vi "Case Structure Tunnels.vi"   [LabVIEW 2015]
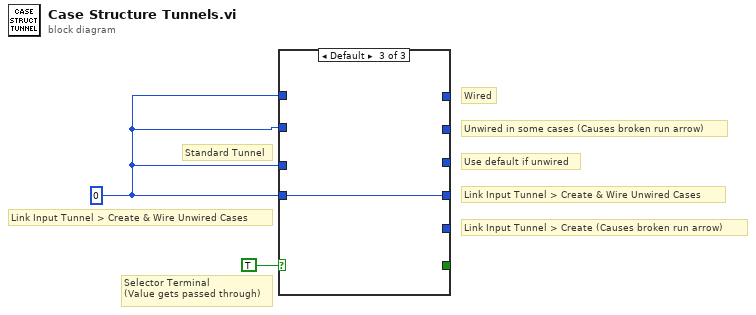
[diagram p0: block diagram]
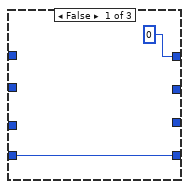
[diagram p2: hidden frame]
diagram:
  w1 = 0
  # "Standard Tunnel"
  # "Link Input Tunnel > Create & Wire Unwired Cases"
  # "Selector Terminal\n(Value gets passed through)"
  # "Link Input Tunnel > Create (Causes broken run arrow)"
  # "Link Input Tunnel > Create & Wire Unwired Cases"
  # "Wired"
  # "Use default if unwired"
  # "Unwired in some cases (Causes broken run arrow)"
  n1 = case TRUE {
    selector: TRUE -> [_ w5 _]
    tunnel: [_ w6 _] -> _
    tunnel: [_ w6 _] -> _
    tunnel: [w3 w6 w7] -> _
    tunnel: [_ w6 _] -> _
    tunnel: [0 w6 _] -> _
    tunnel: w1 -> [_ _ _]
    tunnel: w1 -> [_ _ _]
    tunnel: [_ w5 _] -> _
    tunnel: w1 -> [_ _ _]
    tunnel: w1 -> [w3 w6 w7]
    frame False {
    }
    frame True {
    }
    frame Default {
    }
  }
